vi "Get Switch node.vi"(8 "error in (no error)":errorcluster, 10 "Engine":string="Switch", 11 "DMM Instrument":refnum<class "DMM Instrument.lvclass">) -> (0 "error out":errorcluster, 2 "Switch node":refnum<data-value>, 3 "DMM Instrument out":refnum<class "DMM Instrument.lvclass">)   [LabVIEW 2025]
uses:
  DMM Instrument.lvclass
  C:/Users/Public/Documents/Sandia National Labs/TSS Plugin/CEF.lvlibp/Node/CEF_Node.lvclass
  Users/Public/Documents/Sandia National Labs/TSS Plugin/Abstract Engine.lvlibp/Plugin/Abstract/Abstract Instrument/Abstract Instrument.lvclass
  SwitchDMM Channel/SwitchDMM Channel.lvclass
  SwitchDMM Channel configuration/SwitchDMM Channel configuration.lvclass
  SwitchDMM Channel configuration/SwitchDMM Channel configuration.lvclass/SwitchDMM Channel configuration.ctl
  SwitchDMM Channel configuration/Read SwitchDMM Channel.vi
  Users/Public/Documents/Sandia National Labs/TSS Plugin/CEF.lvlibp/Node/ReadChildren.vi
  Users/Public/Documents/Sandia National Labs/TSS Plugin/CEF.lvlibp/Node/ReadParent.vi
  Users/Public/Documents/Sandia National Labs/TSS Plugin/CEF.lvlibp/Node/CEF_Node.lvclass
  Users/Public/Documents/Sandia National Labs/TSS Plugin/CEF.lvlibp/serializable configuration/CEF_serializable configuration.lvclass
  DMM Instrument.lvclass/DMM Instrument.ctl
  Users/Public/Documents/Sandia National Labs/TSS Plugin/Abstract Engine.lvlibp/Plugin/Abstract/Abstract Engine/Abstract Engine.lvclass
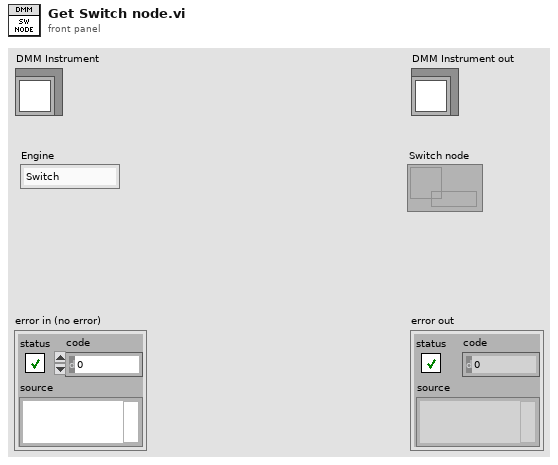
[diagram p1: front panel]
types:
  T1 = typedef "SwitchDMM Channel configuration.lvclass/SwitchDMM Channel.ctl" = cluster{"Switch":string}
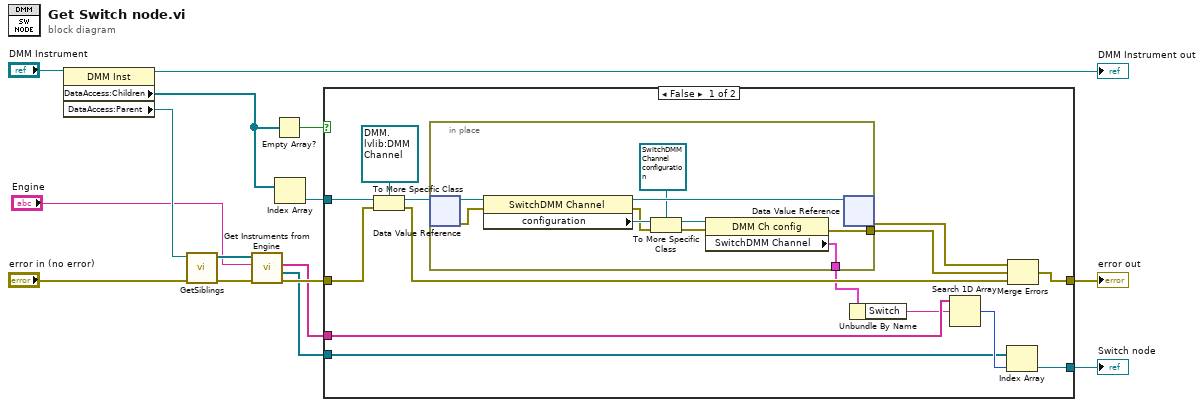
[diagram p0: block diagram]
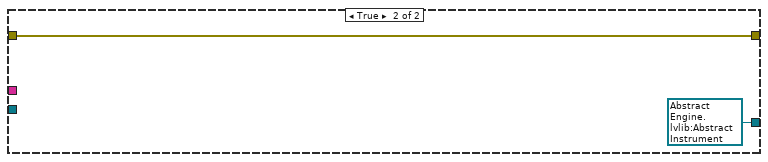
[diagram p2: hidden frame]
diagram:
  n1 = property class="DMM Inst"(reference="DMM Instrument") -> (reference out=→"DMM Instrument out":refnum<class "DMM Instrument.lvclass">, "DataAccess:Children"=w14:refnum<data-value>[], "DataAccess:Parent"=w4:refnum<data-value>)  [unwired: 1 in, 1 out]
  n2 = call "GetSiblings.vi"("error in"="error in (no error)", "node in"=w4) -> ("error out"=w2:errorcluster, "siblings"=w3:refnum<data-value>[])  [unwired: 8 in]
  n3 = call "Get Instruments from Engine.vi"("error in"=w2, "Engine"="Engine", "Engines"=w3) -> ("error out"=w9:errorcluster, "Instrument nodes"=w7:refnum<data-value>[], "Instruments"=w8:string[])  [unwired: 6 in]
  n4 = Empty Array?(array=w14) -> (empty?=w13:bool)
  n5 = Index Array(array=w14) -> (element=w11:refnum<data-value>)  [unwired: 1 in]
  n6 = case shown="False" w13 {
    tunnel: w8 -> [w26 _]
    tunnel: w7 -> [w25 _]
    tunnel: [w24 refnum<data-value> refnum ("target class")] -> w12
    tunnel: w9 -> [w22 w40]
    tunnel: w11 -> [w23 _]
    tunnel: [w19 w40] -> w10
    frame False {
      n7 = To More Specific Class(target class=refnum<data-value> refnum, reference=w23, error in=w22) -> (specific class reference=w28:refnum<data-value>, error out=w21:errorcluster)
      n8 = in-place {
        in-place-border: [w31] -> w20
        in-place-border: [w30] -> w17
        n9 = in-place-dvr #1(w28) -> (w39:refnum<class "SwitchDMM Channel.lvclass">, w34:errorcluster)
        n10 = property class="SwitchDMM Channel"(reference=w39, error in=w34) -> (reference out=w38:refnum<class "SwitchDMM Channel.lvclass">, error out=w33:errorcluster, "configuration"=w37:refnum<class "CEF_serializable configuration.lvclass">)
        n11 = To More Specific Class(target class=refnum<class "SwitchDMM Channel configuration.lvclass"> refnum ("DMM.lvlib:DMM Ch config"), reference=w37, error in=w33) -> (specific class reference=w36:refnum<class "SwitchDMM Channel configuration.lvclass">, error out=w32:errorcluster)
        n12 = property class="DMM Ch config"(reference=w36, error in=w32) -> (error out=w31:errorcluster, "SwitchDMM Channel"=w30:T1)  [unwired: 1 out]
        n13 = in-place-dvr #1(w38) -> (w18:errorcluster)  [unwired: 1 out]
      }
      n14 = Unbundle By Name(w17) -> ("Switch"=w16:string)
      n15 = Search 1D Array(1D array=w26, element=w16) -> (index of element=w27:i32)  [unwired: 1 in]
      n16 = Index Array(array=w25, index=w27) -> (element=w24:refnum<data-value>)
      n17 = Merge Errors(w18, w20, w21) -> (w19:errorcluster)
    }
    frame True {
    }
  }
  "error out" <- w10
  "Switch node" <- w12
